vi "Register gRPC Methods.vi"(8 "error in (no error)":errorcluster, 11 "Template Server in":refnum<class "MeasurementService.lvclass">) -> (0 "error out":errorcluster, 3 "Template Server out":refnum<class "MeasurementService.lvclass">)   [LabVIEW 2020, in "CancellableMeasurementProxy.lvlib" / "MeasurementService.lvclass"]
uses:
  MeasurementService.lvclass
  typeDefs/Server Internal UEs.ctl
  typeDefs/Server Internal Message.ctl
  typeDefs/Server gRPC UEs.ctl
  <vilib>/gRPC/LabVIEW gRPC Library/Server API/typeDefs/gRPCId Cluster.ctl
  <vilib>/gRPC/LabVIEW gRPC Library/Shared/grpcId.ctl
  MeasurementService.lvclass/MeasurementService.ctl
  <vilib>/gRPC/LabVIEW gRPC Library/grpc-lvsupport-release.lvlib
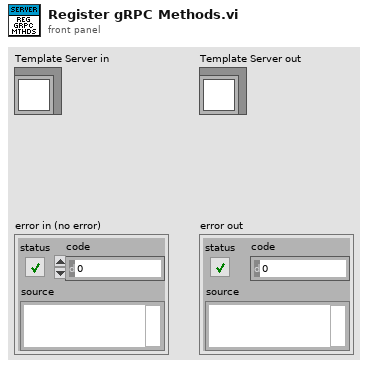
[diagram p1: front panel]
types:
  T1 = typedef "CancellableMeasurementProxy.lvlib/MeasurementService.lvclass/Server gRPC UEs.ctl" = cluster{"MeasurementService GetMetadata gRPC UE":refnum<user-event>, "MeasurementService Measure gRPC UE":refnum<user-event>}
  T2 = typedef "CancellableMeasurementProxy.lvlib/MeasurementService.lvclass/Server Internal UEs.ctl" = cluster{"MeasurementService GetMetadata Internal UE":refnum<user-event>, "MeasurementService Measure Internal UE":refnum<user-event>}
  T3 = typedef "grpc-lvsupport-release.lvlib/grpcId.ctl" = u64
  T4 = typedef "CancellableMeasurementProxy.lvlib/MeasurementService.lvclass/Server Internal Message UE.ctl" = refnum<user-event>
  T5 = typedef "grpc-lvsupport-release.lvlib/gRPCId Cluster UE.ctl" = refnum<user-event>
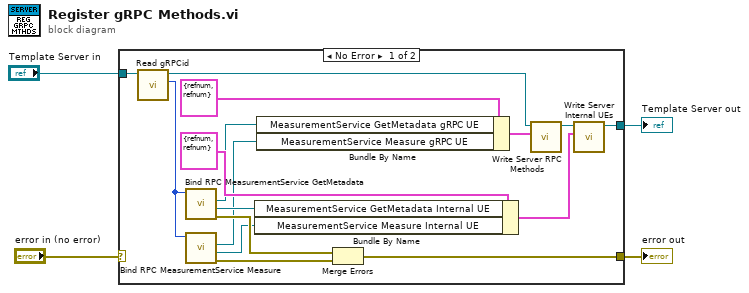
[diagram p0: block diagram]
diagram:
  n1 = case shown="No Error" "error in (no error)" {
    selector: "error in (no error)" -> [_ w21]
    tunnel: "Template Server in" -> [w12 w22]
    tunnel: [w20 w21] -> w3
    tunnel: [w19 w22] -> w2
    frame No Error {
      n2 = call-dynamic "Read gRPCid.vi"("iService in"=w12) -> ("gRPCid"=w11:T3, "iService out"=w13:refnum<class "MeasurementService.lvclass">)  [unwired: 8 in, 1 out]
      n3 = call "Bind RPC MeasurementService GetMetadata.vi"("gRPCid server in"=w11) -> ("error out"=w10:errorcluster, "MeasurementService GetMetadata Internal UE"=w8:T4, "MeasurementService GetMetadata gRPC UE"=w9:T5)  [unwired: 7 in, 1 out]
      n4 = call "Bind RPC MeasurementService Measure.vi"("gRPCid server in"=w11) -> ("error out"=w7:errorcluster, "MeasurementService Measure Internal UE"=w5:T4, "MeasurementService Measure gRPC UE"=w6:T5)  [unwired: 7 in, 1 out]
      n5 = Bundle By Name ("Bundle Internal UEs")(cluster=T2 {"MeasurementService GetMetadata Internal UE"=refnum, "MeasurementService Measure Internal UE"=refnum} ("Server Internal UEs"), "MeasurementService GetMetadata Internal UE"=w8, "MeasurementService Measure Internal UE"=w5) -> (w18:T2)
      n6 = Bundle By Name ("Bundle gRPC UEs")(cluster=T1 {"MeasurementService GetMetadata gRPC UE"=refnum, "MeasurementService Measure gRPC UE"=refnum} ("gRPC Server Method Events"), "MeasurementService GetMetadata gRPC UE"=w9, "MeasurementService Measure gRPC UE"=w6) -> (w15:T1)
      n7 = Merge Errors(w10, w7) -> (w20:errorcluster)
      n8 = call "Write Server RPC Methods.vi"("Server RPC Methods"=w15, "SignalGeneratorService in"=w13) -> ("SignalGeneratorService out"=w16:refnum<class "MeasurementService.lvclass">)  [unwired: 8 in, 1 out]
      n9 = call "Write Server Internal UEs.vi"("Server Internal UEs"=w18, "SignalGeneratorService in"=w16) -> ("SignalGeneratorService out"=w19:refnum<class "MeasurementService.lvclass">)  [unwired: 8 in, 1 out]
    }
    frame Error {
    }
  }
  "error out" <- w3
  "Template Server out" <- w2
